vi "Get ANN outputs.vi"(1 "1D ANN config":i32[](array[numeric]), 2 "Neurons ouputs":dbl[][](array[numeric]) format="%.2f") -> (0 "ANN outputs":dbl[](array[numeric]) format="%.2f")   [LabVIEW 2010]
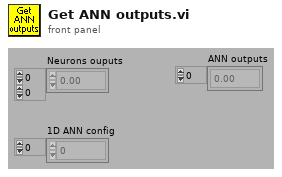
[diagram p1: front panel]
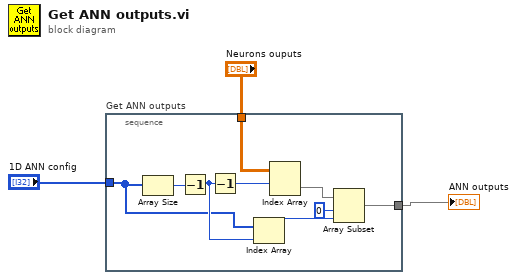
[diagram p0: block diagram]
diagram:
  n1 = stacked-sequence "Get ANN outputs" {
    tunnel: "1D ANN config" -> [w11]
    tunnel: [w9] -> w2
    tunnel: "Neurons ouputs" -> [w5]
    frame #0 {
      n2 = Array Size(array=w11) -> (size(s)=w4:i32)
      n3 = Decrement(x=w4) -> (x-1=w12:i32)
      n4 = Decrement(x=w12) -> (x-1=w6:i32)
      n5 = Index Array(array=w11, index=w12) -> (element=w10:i32)
      n6 = Index Array(array=w5, index (row)=w6) -> (element=w7:dbl[])  [unwired: 1 in]
      n7 = Array Subset(array=w7, index=0 ("Array Index"), length=w10) -> (w9:dbl[])
    }
  }
  "ANN outputs" <- w2
